vi "Stop Acquisition.vi"(8 "error in (no error)":errorcluster, 11 "IMAQdx Cam Actor in":refnum<class "IMAQdx Cam Actor.lvclass">) -> (0 "error out":errorcluster, 3 "IMAQdx Cam Actor out":refnum<class "IMAQdx Cam Actor.lvclass">)   [LabVIEW 2014, in "IMAQdx Cam Actor.lvlib" / "IMAQdx Cam Actor.lvclass"]
uses:
  IMAQdx Cam Actor.lvclass
  <vilib>/userdefined/High Color/IMAQdx.ctl
  IMAQdx Cam Actor.lvclass/IMAQdx Cam Actor.ctl
  <vilib>/vision/driver/NI_Vision_Acquisition_Software.lvlib
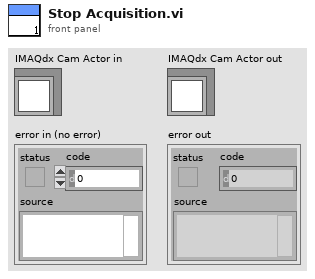
[diagram p1: front panel]
types:
  T1 = typedef "IMAQdx.ctl" = refnum<k21>
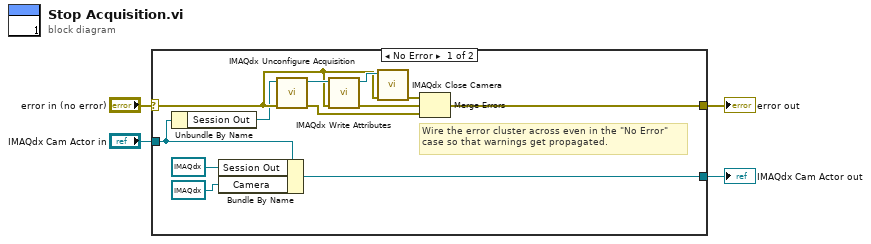
[diagram p0: block diagram]
diagram:
  n1 = case shown="No Error" "error in (no error)" {
    selector: "error in (no error)" -> [w14 w18]
    tunnel: [w10 w18] -> w3
    tunnel: [w7 w17] -> w1
    tunnel: "IMAQdx Cam Actor in" -> [w9 w17]
    frame No Error {
      # "Wire the error cluster across even in the \"No Error\"\ncase so that warnings get propagated."
      n2 = Unbundle By Name(w9) -> ("Session Out"=w8:T1)
      n3 = Bundle By Name(cluster=w9, "Session Out"=T1 refnum, "Camera"=T1 refnum) -> (w7:refnum<class "IMAQdx Cam Actor.lvclass">)
      n4 = call <vilib>:"IMAQdx Unconfigure Acquisition.vi"("error in"=w14, "Session In"=w8) -> ("error out"=w11:errorcluster, "Session Out"=w15:T1)  [unwired: 8 out]
      n5 = call <vilib>:"IMAQdx Write Attributes.vi"("error in"=w14, "Session In"=w15) -> ("error out"=w12:errorcluster, "Session Out"=w16:T1)  [unwired: 8 in]
      n6 = call <vilib>:"IMAQdx Close Camera.vi"("error in"=w14, "Session In"=w16) -> ("error out"=w13:errorcluster)  [unwired: 9 out]
      n7 = Merge Errors(w13, w12, w11) -> (w10:errorcluster)
    }
    frame Error {
    }
  }
  "error out" <- w3
  "IMAQdx Cam Actor out" <- w1
